vi "Create sine wave for generation.vi"() -> ()   [LabVIEW 2019]
uses:
  <vilib>/measure/matone.llb/Extract Single Tone Information 1 Chan.vi
  <vilib>/Analysis/NI_AALBase.lvlib
  <vilib>/measure/NI_MAPro.lvlib
panel:
  in  "cycles":dbl=10.0
  out "detected frequency":dbl format="%.2p"
  out "size(s)":i32
  out "signal":waveform(dbl)(graph)
  in  "sampling info":cluster{"Fs":dbl, "#s":dbl}={"Fs"=3072000000.0, "#s"=160000.0}
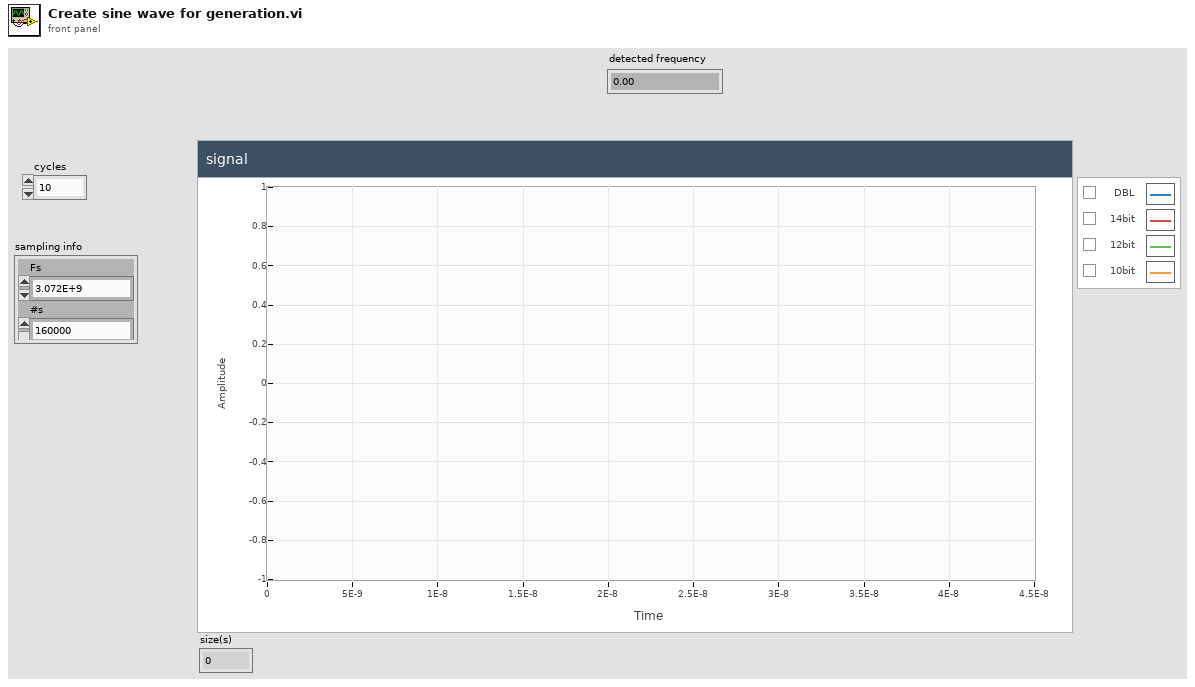
[diagram p1: front panel]
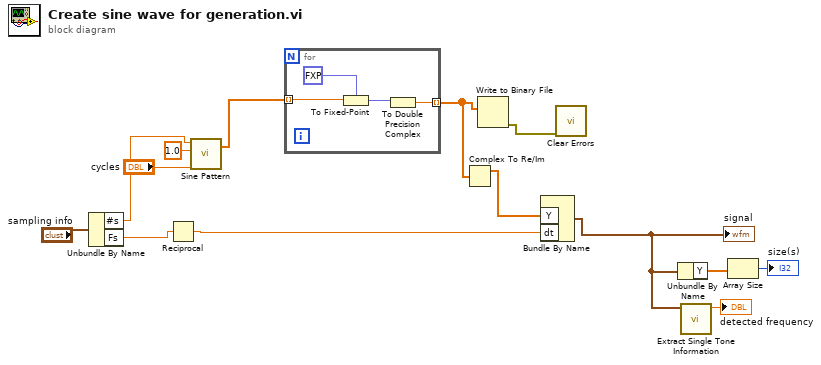
[diagram p0: block diagram]
diagram:
  n1 = Unbundle By Name("sampling info") -> ("#s"=w9:dbl, "Fs"=w11:dbl)
  n2 = Reciprocal(x=w11) -> (1/x=w10:dbl)
  n3 = call <vilib>:"Sine Pattern.vi"("cycles"="cycles", "amplitude"=1.0, "samples"=w9) -> ("Sinusoidal Pattern"=w4:dbl[])  [unwired: 1 in, 1 out]
  n4 = for {
    tunnel: w4 -> [w18] mode=indexing
    tunnel: [w15] -> w2 mode=indexing
    n5 = To Fixed-Point(fixed-point type=fxp<+/-,14,1> 0.0, number=w18) -> (fixed-point=w16:fxp<+/-,14,1>)
    n6 = To Double Precision Complex(1:w16) -> (0:w15:cdb)
  }
  n7 = Complex To Re/Im(x + iy=w2) -> (x=w1:dbl[])  [unwired: 1 out]
  n8 = Write to Binary File(data=w2) -> (error out=w3:errorcluster)  [unwired: 5 in, 2 out]
  n9 = Bundle By Name("Y"=w1, "dt"=w10) -> (w7:waveform(dbl))  [unwired: 1 in]
  "signal" <- w7
  n10 = call <vilib>:"Clear Errors.vi"("error in (no error)"=w3) -> ()  [unwired: 5 in, 2 out]
  n11 = Unbundle By Name(w7) -> ("Y"=w8:dbl[])
  n12 = call-poly <vilib>:"Extract Single Tone Information.vi"("time signal in"=w7) -> ("detected frequency"=→"detected frequency":dbl)  [unwired: 5 in, 5 out]
  n13 = Array Size(array=w8) -> (size(s)=→"size(s)":i32)
